vi "極限逃脫Top.vi"() -> ()   [LabVIEW 2014]
panel:
  in  "stop":bool
  in  "Cluster":T1
  # "極限逃脫"
  # "1"
  # "2"
  # "4"
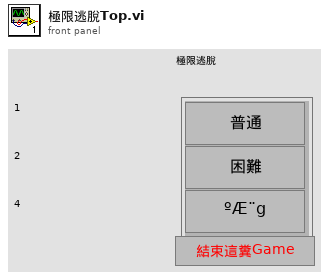
[diagram p1: front panel]
types:
  T1 = cluster{"OK Button":bool, "OK Button 2":bool, "OK Button 3":bool}
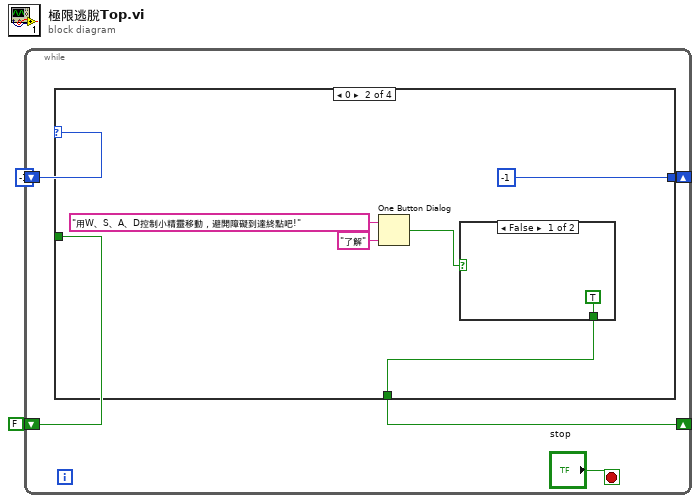
[diagram p0: block diagram]
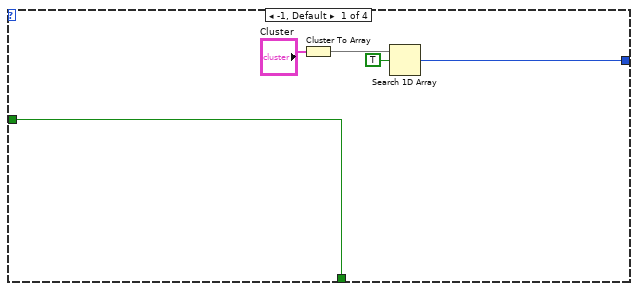
[diagram p2: hidden frame]
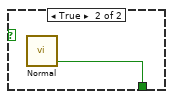
[diagram p3: hidden frame]
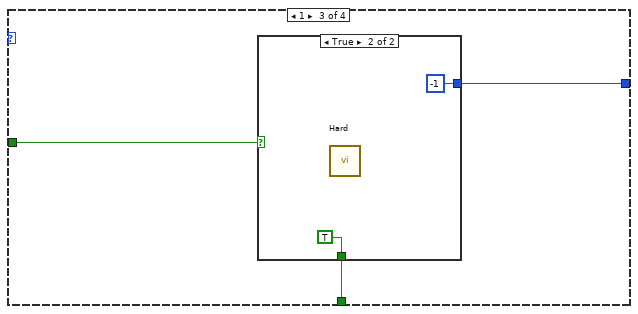
[diagram p4: hidden frame]
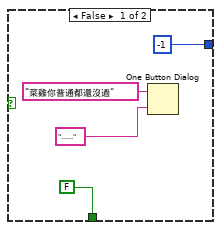
[diagram p5: hidden frame]
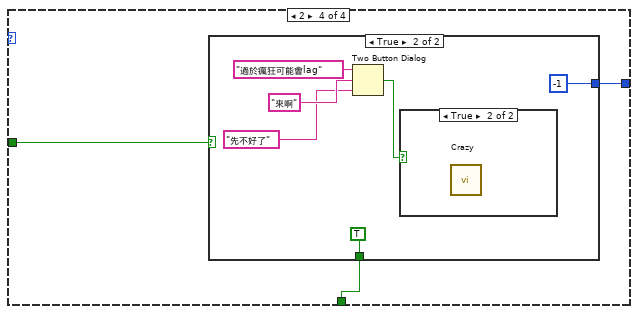
[diagram p6: hidden frame]
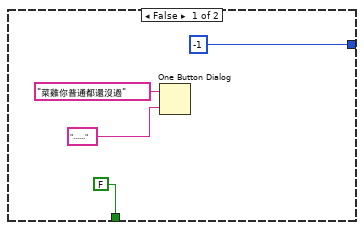
[diagram p7: hidden frame]
diagram:
  n1 = while {
    shift-right: [w5] -> _
    shift-left: FALSE -> [w6]
    shift-right: [w4] -> _
    shift-left: -1 ("index of element") -> [w3]
    stop <- "stop" stop-if-true
    n2 = case shown="0" w3 {
      tunnel: [w8 w15 w21 w30] -> w5
      tunnel: w6 -> [w8 _ w22 w31]
      tunnel: [w9 -1 ("index of element") w20 w29] -> w4
      frame -1, Default {
        n3 = Cluster To Array(cluster="Cluster") -> (array=w11:bool[])
        n4 = Search 1D Array(1D array=w11, element=TRUE) -> (index of element=w9:i32)  [unwired: 1 in]
      }
      frame 0 {
        n5 = One Button Dialog(message="用W、S、A、D控制小精靈移動，避開障礙到達終點吧!", button name ("OK")="了解") -> (true=w16:bool)
        n6 = case shown="False" w16 {
          tunnel: [TRUE ("高難度挑戰") w19] -> w15
          frame False {
          }
          frame True {
            n7 = call "Normal.vi"() -> ("高難度挑戰"=w19:bool)  [unwired: 5 in]
          }
        }
      }
      frame 1 {
        n8 = case shown="True" w22 {
          tunnel: [FALSE TRUE] -> w21
          tunnel: [-1 ("index of element") -1 ("index of element")] -> w20
          frame False {
            n9 = One Button Dialog(message="菜雞你普通都還沒過", button name ("OK")="......") -> ()  [unwired: 1 out]
          }
          frame True {
            n10 = call "Hard.vi"() -> ()  [unwired: 6 in]
          }
        }
      }
      frame 2 {
        n11 = case shown="True" w31 {
          tunnel: [FALSE TRUE] -> w30
          tunnel: [-1 ("index of element") -1 ("index of element")] -> w29
          frame False {
            n12 = One Button Dialog(message="菜雞你普通都還沒過", button name ("OK")="......") -> ()  [unwired: 1 out]
          }
          frame True {
            n13 = Two Button Dialog(message="過於瘋狂可能會lag", 1:"先不好了" ("F button name (\"Cancel\")"), 2:"來啊" ("T button name (\"OK\")")) -> (T button?=w39:bool)
            n14 = case shown="True" w39 {
              frame False {
              }
              frame True {
                n15 = call "Crazy.vi"() -> ()  [unwired: 6 in]
              }
            }
          }
        }
      }
    }
  }
